vi "round to nearest half integer.vi"(1 "Numeric":dbl format="%#_13g") -> (0 "rounded to nearest 0.5":dbl)   [LabVIEW 2016]
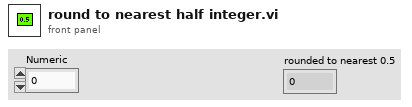
[diagram p1: front panel]
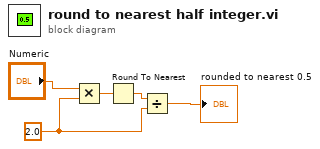
[diagram p0: block diagram]
diagram:
  w2 = 2.0 ("y")
  n1 = Multiply(x="Numeric", y=w2) -> (x*y=w4:dbl)
  n2 = Round To Nearest(number=w4) -> (nearest integer value=w3:dbl)
  n3 = Divide(x=w3, y=w2) -> (x/y=→"rounded to nearest 0.5":dbl)
